vi "Conversao_valores_UCM.0300_SAIDA.vi"(11 "UCM.004.EEL.0300_SAIDA(Controle)":T2) -> (3 "UCM.004.EEL.0300_SAIDA(Indicador)":T2)   [LabVIEW 2019]
uses:
  padrao_UCM.004.EEL.0300_SAIDA.ctl
panel:
  in  "ANALOGICO_saida":T1
  out "ANALOGICO_entrada":T1
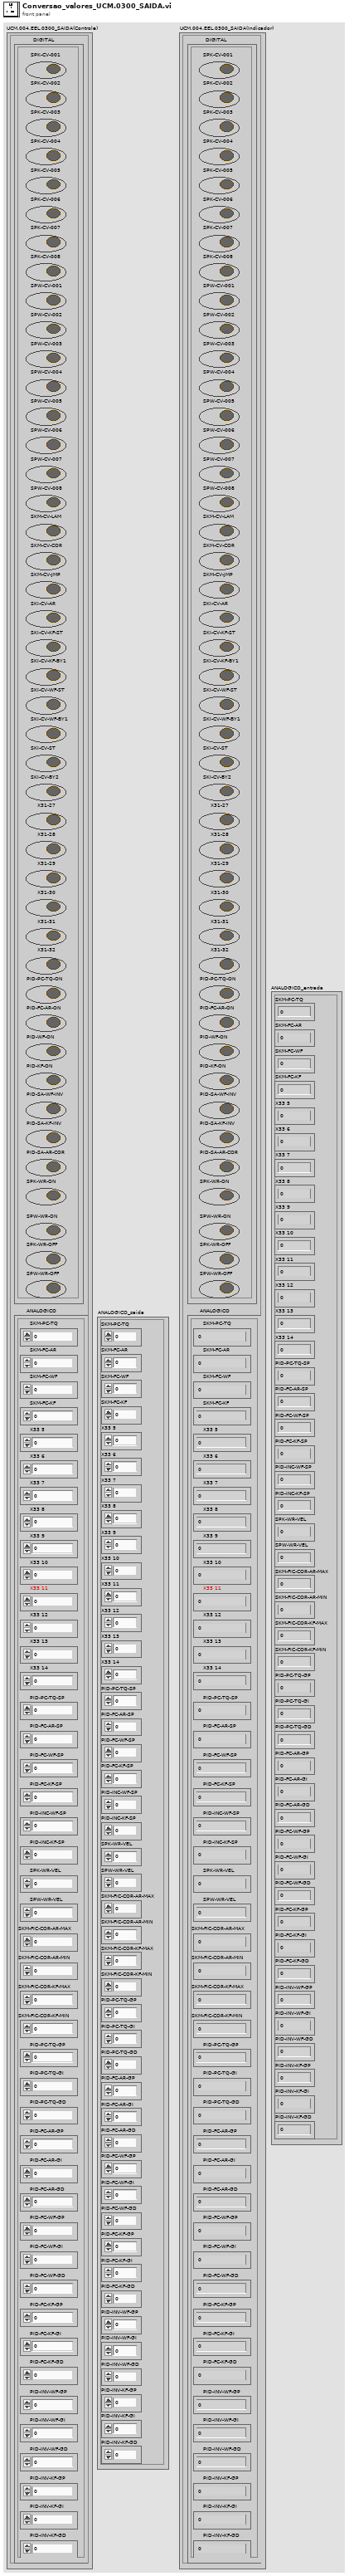
[diagram p1: front panel]
types:
  T1 = cluster{"SKM-PC-TQ":i16, "SKM-FC-AR":i16, "SKM-FC-WF":i16, "SKM-FC-KF":i16, "X33 5":i16, "X33 6":i16, "X33 7":i16, "X33 8":i16, "X33 9":i16, "X33 10":i16, "X33 11":i16, "X33 12":i16, "X33 13":i16, "X33 14":i16, "PID-PC-TQ-SP":i16, "PID-FC-AR-SP":i16, "PID-FC-WF-SP":i16, "PID-FC-KF-SP":i16, "PID-INC-WF-SP":i16, "PID-INC-KF-SP":i16, "SPK-WR-VEL":i32, "SPW-WR-VEL":i32, "SKM-FIC-COR-AR-MAX":dbl, "SKM-FIC-COR-AR-MIN":dbl, "SKM-FIC-COR-KF-MAX":dbl, "SKM-FIC-COR-KF-MIN":dbl, "PID-PC-TQ-GP":dbl, "PID-PC-TQ-GI":dbl, "PID-PC-TQ-GD":dbl, "PID-FC-AR-GP":dbl, "PID-FC-AR-GI":dbl, "PID-FC-AR-GD":dbl, "PID-FC-WF-GP":dbl, "PID-FC-WF-GI":dbl, "PID-FC-WF-GD":dbl, "PID-FC-KF-GP":dbl, "PID-FC-KF-GI":dbl, "PID-FC-KF-GD":dbl, "PID-INV-WF-GP":dbl, "PID-INV-WF-GI":dbl, "PID-INV-WF-GD":dbl, "PID-INV-KF-GP":dbl, "PID-INV-KF-GI":dbl, "PID-INV-KF-GD":dbl}
  T2 = typedef "padrao_UCM.004.EEL.0300_SAIDA.ctl" = cluster{"DIGITAL":cluster{"SPK-CV-001":bool, "SPK-CV-002":bool, "SPK-CV-003":bool, "SPK-CV-004":bool, "SPK-CV-005":bool, "SPK-CV-006":bool, "SPK-CV-007":bool, "SPK-CV-008":bool, "SPW-CV-001":bool, "SPW-CV-002":bool, "SPW-CV-003":bool, "SPW-CV-004":bool, "SPW-CV-005":bool, "SPW-CV-006":bool, "SPW-CV-007":bool, "SPW-CV-008":bool, "SKM-CV-LAM":bool, "SKM-CV-COR":bool, "SKM-CV-JMP":bool, "SKI-CV-AR":bool, "SKI-CV-KF-ST":bool, "SKI-CV-KF-BY1":bool, "SKI-CV-WF-ST":bool, "SKI-CV-WF-BY1":bool, "SKI-CV-ST":bool, "SKI-CV-BY2":bool, "X31-27":bool, "X31-28":bool, "X31-29":bool, "X31-30":bool, "X31-31":bool, "X31-32":bool, "PID-PC-TQ-ON":bool, "PID-FC-AR-ON":bool, "PID-WF-ON":bool, "PID-KF-ON":bool, "PID-SA-WF-INV":bool, "PID-SA-KF-INV":bool, "PID-SA-AR-COR":bool, "SPK-WR-ON":bool, "SPW-WR-ON":bool, "SPK-WR-OFF":bool, "SPW-WR-OFF":bool}, "ANALOGICO":cluster{"SKM-PC-TQ":i16, "SKM-FC-AR":i16, "SKM-FC-WF":i16, "SKM-FC-KF":i16, "X33 5":i16, "X33 6":i16, "X33 7":i16, "X33 8":i16, "X33 9":i16, "X33 10":i16, "X33 11":i16, "X33 12":i16, "X33 13":i16, "X33 14":i16, "PID-PC-TQ-SP":i16, "PID-FC-AR-SP":i16, "PID-FC-WF-SP":i16, "PID-FC-KF-SP":i16, "PID-INC-WF-SP":i16, "PID-INC-KF-SP":i16, "SPK-WR-VEL":i32, "SPW-WR-VEL":i32, "SKM-FIC-COR-AR-MAX":dbl, "SKM-FIC-COR-AR-MIN":dbl, "SKM-FIC-COR-KF-MAX":dbl, "SKM-FIC-COR-KF-MIN":dbl, "PID-PC-TQ-GP":dbl, "PID-PC-TQ-GI":dbl, "PID-PC-TQ-GD":dbl, "PID-FC-AR-GP":dbl, "PID-FC-AR-GI":dbl, "PID-FC-AR-GD":dbl, "PID-FC-WF-GP":dbl, "PID-FC-WF-GI":dbl, "PID-FC-WF-GD":dbl, "PID-FC-KF-GP":dbl, "PID-FC-KF-GI":dbl, "PID-FC-KF-GD":dbl, "PID-INV-WF-GP":dbl, "PID-INV-WF-GI":dbl, "PID-INV-WF-GD":dbl, "PID-INV-KF-GP":dbl, "PID-INV-KF-GI":dbl, "PID-INV-KF-GD":dbl}}
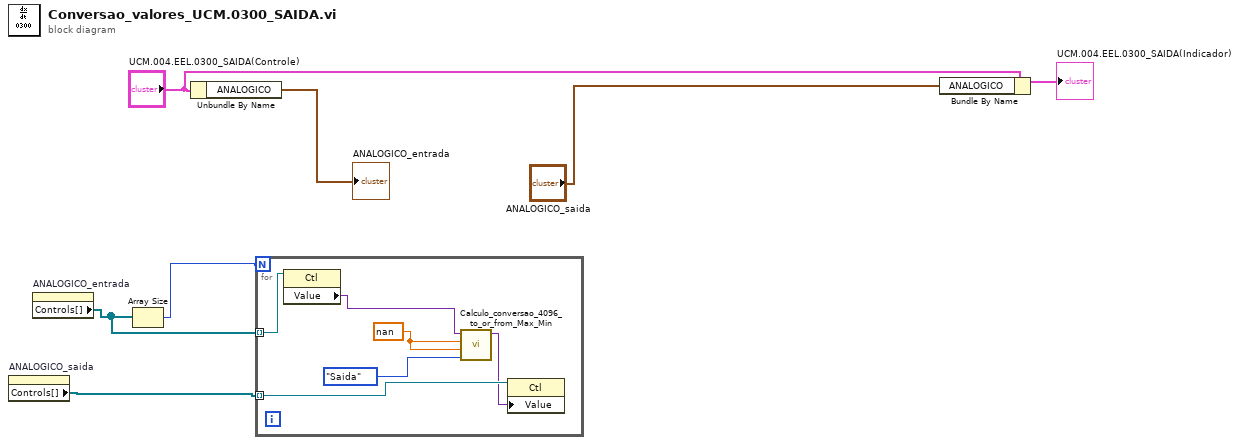
[diagram p0: block diagram]
diagram:
  n1 = property on="ANALOGICO_saida" class="Clust (strict)"() -> ("Controls[]"=w2:refnum<vi>[])  [unwired: 2 in, 2 out]
  n2 = property on="ANALOGICO_entrada" class="Clust (strict)"() -> ("Controls[]"=w3:refnum<vi>[])  [unwired: 2 in, 2 out]
  n3 = Array Size(array=w3) -> (size(s)=w5:i32)
  n4 = Unbundle By Name("UCM.004.EEL.0300_SAIDA(Controle)") -> ("ANALOGICO"=→"ANALOGICO_entrada":T1)
  n5 = for {
    N: w5 -> [_]
    tunnel: w2 -> [w13] mode=indexing
    tunnel: w3 -> [w8] mode=indexing
    w11 = nan
    n6 = property class="Ctl"(reference=w8) -> ("Value"=w9:variant)  [unwired: 1 in, 2 out]
    n7 = call "Calculo_conversao_4096_to_or_from_Max_Min.vi"("Tipo"=enum16{"Saida", "Entrada"}."Saida", "Min"=w11, "Max"=w11, "Value"=w9) -> ("Value 2"=w10:variant)  [unwired: 7 in]
    n8 = property class="Ctl"(reference=w13, "Value"=w10) -> ()  [unwired: 1 in, 2 out]
  }
  n9 = Bundle By Name(cluster="UCM.004.EEL.0300_SAIDA(Controle)", "ANALOGICO"="ANALOGICO_saida") -> (→"UCM.004.EEL.0300_SAIDA(Indicador)":T2)
